vi "Label Targets2.vi"(6 "Edges":cluster{"X":sgl, "Y":sgl}[](array[cluster]), 8 "Line":T1, 9 "Annotate":bool=TRUE, 10 "Results":T3 {"Score" format="%#_3g"; "Pixels"."Rectangle"."Numeric 5" format="%#_3g"; "Pixels"."Rectangle"."Numeric 3" format="%#_3g"; "Pixels"."Rectangle"."Numeric 2" format="%#_3g"; "Pixels"."Rectangle"."Numeric" format="%#_3g"; "Normalized"."Rectangle"."Numeric 5" format="%#_2g"; "Normalized"."Rectangle"."Numeric 3" format="%#_2g"; "Normalized"."Rectangle"."Numeric 2" format="%#_2g"; "Normalized"."Rectangle"."Numeric" format="%#_2g"; "Normalized"."Center"."?" format="%#_3g"; "Normalized"."Center"."?" format="%#_3g"; "Distance (ft)" format="%#_3g"}, 11 "Image in":T2) -> (3 "Image out":T2)   [LabVIEW 2016]
doc: "Draw text values near or on the particle and draws a square around the target stripes.."
uses:
  <vilib>/vision/Image Controls.llb/IMAQ Image.ctl
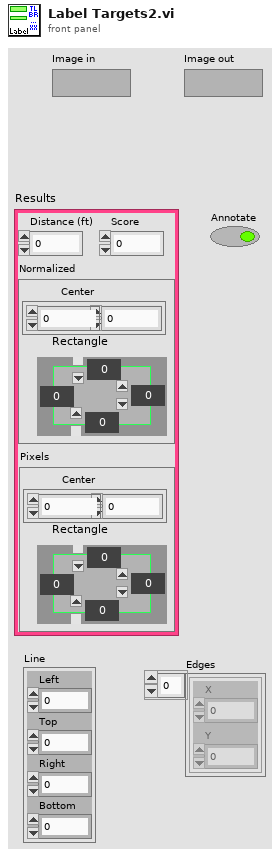
[diagram p1: front panel]
types:
  T1 = cluster{"Left":dbl, "Top":dbl, "Right":dbl, "Bottom":dbl}
  T2 = typedef "IMAQ Image.ctl" = refnum<image>
  T3 = cluster{"Distance (ft)":dbl, "Score":dbl, "Normalized":cluster{"Center":cluster{dbl, dbl}, "Rectangle":cluster{"Numeric":dbl, "Numeric 2":dbl, "Numeric 3":dbl, "Numeric 5":dbl}}, "Pixels":cluster{"Center":cluster{dbl, dbl}, "Rectangle":cluster{"Numeric":dbl, "Numeric 2":dbl, "Numeric 3":dbl, "Numeric 5":dbl}}}
  T4 = cluster{"Desired Font (Application)":enum16{"User-specified Font", "Application Font", "System Font", "Dialog Font"}, "[User-specified Font]":cluster{"Font Name":string, "Size":i16, "Strikeout?":bool, "Italic?":bool, "Underline?":bool, "Outline?":bool, "Shadow?":bool, "Bold?":bool, "Rotation Angle":dbl}, "Horizontal Alignment":i16, "Vertical Alignment":i16}
  T5 = cluster{"Center":cluster{dbl, dbl}, "Rectangle":cluster{"Numeric":dbl, "Numeric 2":dbl, "Numeric 3":dbl, "Numeric 5":dbl}}
  T6 = cluster{"Numeric":dbl, "Numeric 2":dbl, "Numeric 3":dbl, "Numeric 5":dbl}
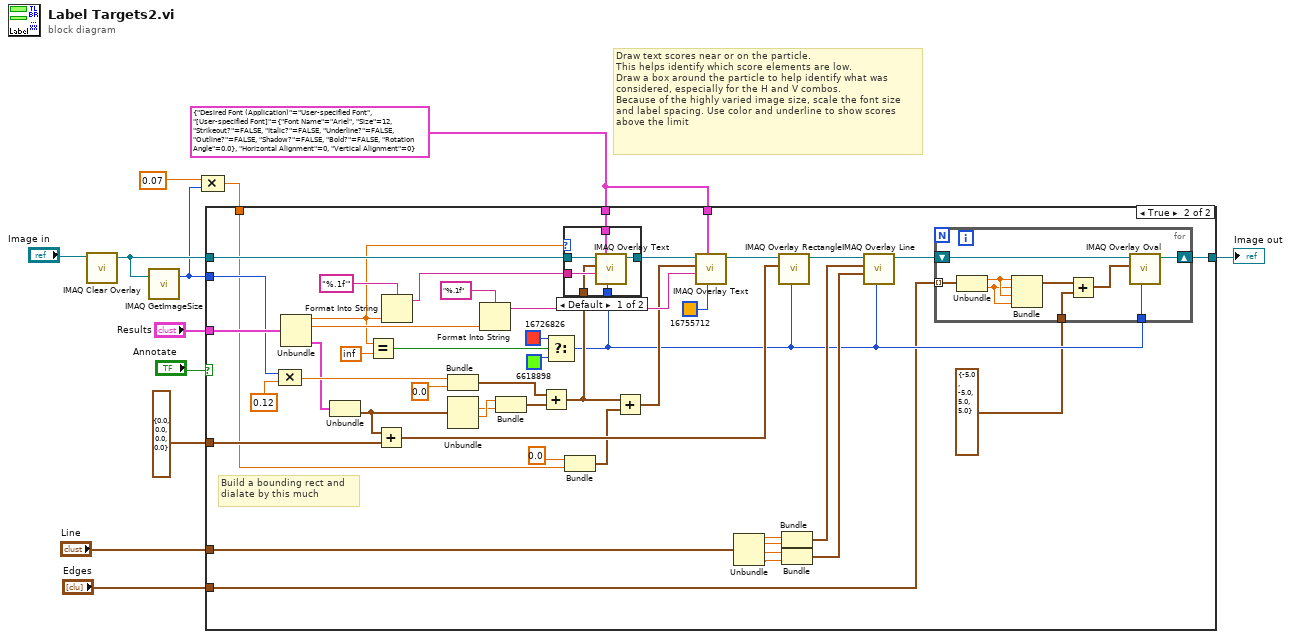
[diagram p0: block diagram]
diagram:
  w1 = T4 {"Desired Font (Application)"=enum."User-specified Font", "[User-specified Font]"={"Font Name"="Ariel", "Size"=12, "Strikeout?"=FALSE, "Italic?"=FALSE, "Underline?"=FALSE, "Outline?"=FALSE, "Shadow?"=FALSE, "Bold?"=FALSE, "Rotation Angle"=0.0}, "Horizontal Alignment"=0, "Vertical Alignment"=0} ("Font, Size & Style")
  # "Draw text scores near or on the particle.\nThis helps identify which score elements are low.\nDraw a box around the particle to help identify what was\nconsidered, especially for the H and V combos.\nBecause of the highly varied image size, scale the font size\nand label spacing. Use color and underline to show scores\nabove the limit"
  n1 = call "IMAQ Clear Overlay"("Image"="Image in") -> ("Image Out"=w8:T2)  [unwired: 2 in, 8 out]
  n2 = call "IMAQ GetImageSize"("Image"=w8) -> ("Y Resolution"=w7:i32)  [unwired: 3 in, 2 out]
  n3 = Compound Arithmetic op=MULTIPLY(0.07, w7) -> (w4:dbl)
  n4 = case shown="True" "Annotate" {
    tunnel: [w13 w20] -> w12
    tunnel: "Results" -> [_ w60]
    tunnel: w8 -> [w13 w59]
    tunnel: w7 -> [_ w58]
    tunnel: cluster{dbl, dbl, dbl, dbl} {0.0, 0.0, 0.0, 0.0} ("output cluster") -> [_ w48]
    tunnel: w4 -> [_ w35]
    tunnel: "Line" -> [_ w29]
    tunnel: "Edges" -> [_ w18]
    tunnel: w1 -> [_ w15]
    tunnel: w1 -> [_ w14]
    frame False {
    }
    frame True {
      # "Build a bounding rect and\ndialate by this much"
      n5 = Compound Arithmetic op=MULTIPLY(w58, 0.12) -> (w51:dbl)
      n6 = Unbundle(w60) -> ("Distance (ft)"=w16:dbl, "Score"=w42:dbl, "Pixels"=w46:T5)  [unwired: 1 out]
      n7 = Unbundle(w46) -> ("Rectangle"=w47:T6)  [unwired: 1 out]
      n8 = Equal?(x=w16, y=inf) -> (x = y?=w31:bool)
      n9 = Add(x=w47, y=w48) -> (x+y=w54:cluster{dbl, dbl, dbl, dbl})
      n10 = Format Into String(format string="%.1f'", w16) -> (resulting string=w49:string)  [unwired: 2 in, 1 out]
      n11 = Bundle(w51, 0.0) -> (w53:cluster{dbl, dbl})  [unwired: 1 in]
      n12 = Unbundle(w47) -> ("Numeric 2"=w56:dbl, "Numeric 3"=w57:dbl)  [unwired: 2 out]
      n13 = Format Into String(format string="%.1f", w42) -> (resulting string=w40:string)  [unwired: 2 in, 1 out]
      n14 = Bundle("Numeric 3"=w57, "Numeric 2"=w56) -> (w55:cluster{"Numeric 3":dbl, "Numeric 2":dbl})  [unwired: 1 in]
      n15 = Add(x=w53, y=w55) -> (x+y=w39:cluster{dbl, dbl})
      n16 = Select(t=u32 16726826 ("Color"), s=w31, f=u32 6618898 ("Color")) -> (s? t:f=w19:u32)
      n17 = case shown="Default" w16 {
        tunnel: w59 -> [w66 w67]
        tunnel: w49 -> [w65 _]
        tunnel: [w64 w67] -> w45
        tunnel: w39 -> [w63 _]
        tunnel: w19 -> [w62 _]
        tunnel: w15 -> [w61 _]
        frame Default {
          n18 = call "IMAQ Overlay Text"("Text Color (black)"=w62, "Font, Size & Style"=w61, "String"=w65, "Origin"=w63, "Image"=w66) -> ("Image Out"=w64:T2)  [unwired: 5 in, 1 out]
        }
        frame 0 {
        }
      }
      n19 = Bundle(0.0, w35) -> (w38:cluster{dbl, dbl})  [unwired: 1 in]
      n20 = Add(x=w39, y=w38) -> (x+y=w36:cluster{dbl, dbl})
      n21 = call "IMAQ Overlay Text"("Text Color (black)"=u32 16755712 ("Color"), "Font, Size & Style"=w14, "String"=w40, "Origin"=w36, "Image"=w45) -> ("Image Out"=w44:T2)  [unwired: 5 in, 1 out]
      n22 = Unbundle(w29) -> ("Left"=w28:dbl, "Top"=w27:dbl, "Right"=w26:dbl, "Bottom"=w25:dbl)
      n23 = call "IMAQ Overlay Rectangle"("Color"=w19, "Rectangle"=w54, "Image"=w44) -> ("Image Out"=w24:T2)  [unwired: 7 in, 1 out]
      n24 = Bundle("Left"=w28, "Top"=w27) -> (w23:cluster{"Left":dbl, "Top":dbl})  [unwired: 1 in]
      n25 = Bundle("Right"=w26, "Bottom"=w25) -> (w22:cluster{"Right":dbl, "Bottom":dbl})  [unwired: 1 in]
      n26 = call "IMAQ Overlay Line"("Color"=w19, "End Point"=w22, "Start Point"=w23, "Image"=w24) -> ("Image Out"=w21:T2)  [unwired: 6 in, 1 out]
      n27 = for {
        shift-right: [w75] -> w20
        shift-left: w21 -> [w76]
        tunnel: w19 -> [w74]
        tunnel: w18 -> [w72] mode=indexing
        tunnel: cluster{"X":sgl, "Y":sgl, "X":sgl, "Y":sgl} {"X"=-5.0, "Y"=-5.0, "X"=5.0, "Y"=5.0} ("output cluster") -> [w68]
        n28 = Unbundle(w72) -> ("X"=w71:sgl, "Y"=w70:sgl)
        n29 = Bundle("X"=w71, "Y"=w70, "X"=w71, "Y"=w70) -> (w69:cluster{"X":sgl, "Y":sgl, "X":sgl, "Y":sgl})  [unwired: 1 in]
        n30 = Add(x=w69, y=w68) -> (x+y=w73:cluster{"X":sgl, "Y":sgl, "X":sgl, "Y":sgl})
        n31 = call "IMAQ Overlay Oval"("Color"=w74, "Bounding Rectangle"=w73, "Image"=w76) -> ("Image Out"=w75:T2)  [unwired: 7 in, 1 out]
      }
    }
  }
  "Image out" <- w12
